vi "Waveform Averaging.vi"(0 "2D curv array in":dbl[][](array[numeric]), 1 "array sensor in":dbl[](array[numeric]), 2 "avg wind1":i32, 3 "2D Sw Array In":dbl[][](array[numeric]), 4 "avg Win2":i32) -> (14 "2D curv Array out":dbl[][](array[numeric]), 15 "2D Sw Array Out":dbl[][](array[numeric]), 16 "Curv Average Array Out":dbl[](array[numeric]), 17 "SW Average Array Out":dbl[](array[numeric]))   [LabVIEW 2019]
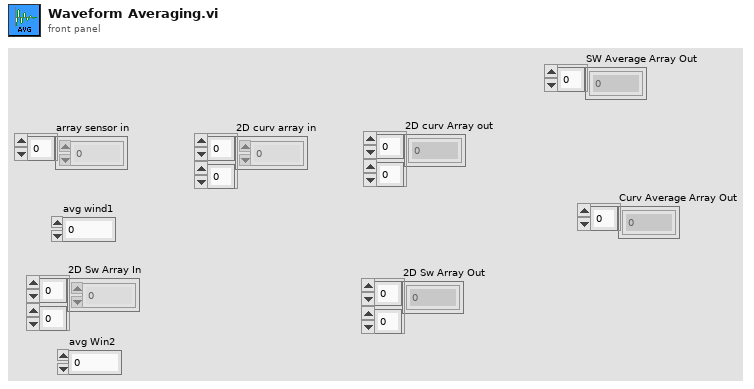
[diagram p1: front panel]
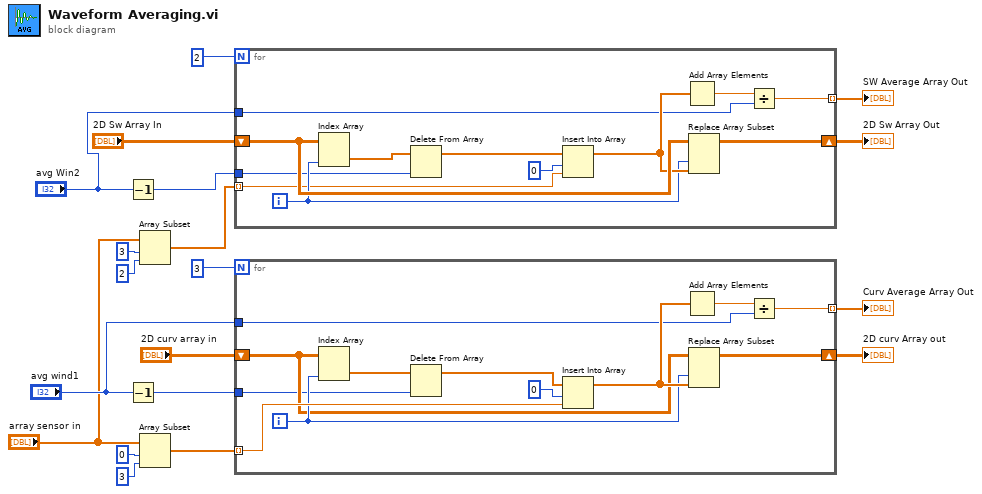
[diagram p0: block diagram]
diagram:
  n1 = Decrement(x="avg Win2") -> (x-1=w18:i32)
  n2 = Decrement(x="avg wind1") -> (x-1=w11:i32)
  n3 = Array Subset(array="array sensor in", index=3, length=2) -> (w2:dbl[])
  n4 = Array Subset(array="array sensor in", index=0, length=3) -> (w12:dbl[])
  n5 = for {
    N: 2 -> [_]
    tunnel: w18 -> [w20]
    tunnel: [w25] -> w7 mode=indexing
    shift-right: [w24] -> w8
    shift-left: "2D Sw Array In" -> [w31]
    tunnel: w2 -> [w22] mode=indexing
    tunnel: "avg Win2" -> [w21]
    i -> [w23]
    n6 = Index Array "Index Array"(array=w31, index (col)=w23) -> (element=w29:dbl[])  [unwired: 1 in]
    n7 = Delete From Array "Delete From Array"(array=w29, index=w20) -> (array with subset deleted=w30:dbl[])  [unwired: 1 in, 1 out]
    n8 = Insert Into Array "Insert Into Array"(array=w30, index=0, new element=w22) -> (w26:dbl[])
    n9 = Add Array Elements(numeric array=w26) -> (sum=w27:dbl)
    n10 = Replace Array Subset "Replace Array Subset"(array=w31, new element=w26, index (col)=w23) -> (w24:dbl[][])  [unwired: 1 in]
    n11 = Divide(x=w27, y=w21) -> (x/y=w25:dbl)
  }
  "2D Sw Array Out" <- w8
  "SW Average Array Out" <- w7
  n12 = for {
    N: 3 -> [_]
    tunnel: w12 -> [w38] mode=indexing
    tunnel: [w37] -> w17 mode=indexing
    shift-right: [w34] -> w9
    shift-left: "2D curv array in" -> [w35]
    tunnel: "avg wind1" -> [w33]
    tunnel: w11 -> [w32]
    i -> [w36]
    n13 = Index Array "Index Array"(array=w35, index (col)=w36) -> (element=w42:dbl[])  [unwired: 1 in]
    n14 = Delete From Array "Delete From Array"(array=w42, index=w32) -> (array with subset deleted=w41:dbl[])  [unwired: 1 in, 1 out]
    n15 = Insert Into Array "Insert Into Array"(array=w41, index=0, new element=w38) -> (w40:dbl[])
    n16 = Add Array Elements(numeric array=w40) -> (sum=w39:dbl)
    n17 = Replace Array Subset "Replace Array Subset"(array=w35, new element=w40, index (col)=w36) -> (w34:dbl[][])  [unwired: 1 in]
    n18 = Divide(x=w39, y=w33) -> (x/y=w37:dbl)
  }
  "2D curv Array out" <- w9
  "Curv Average Array Out" <- w17
